vi "test map utils.vi"() -> (2 "pass?":bool)   [LabVIEW 2019, in "LVCOOOP Tests.lvlib"]
uses:
  LVCOOOP Tests.lvlib
  8b7a900f-a1a1-466e-ab71-210356f2434b.vi
  190aee8e-c763-49bc-a4e3-4cdfa35dd57b.vi
  96190adf-c521-424e-a970-e60fe1e5d14e.vi
  571cc04a-834a-4641-954f-49a22e815eb4.vi
  8aebfca1-6881-489a-a878-9dc2cedf487c.vi
  190aee8e-c763-49bc-a4e3-4cdfa35dd57b.vi/c8492b05-ff29-40b2-a5ff-33168be8e6c9.vi
  190aee8e-c763-49bc-a4e3-4cdfa35dd57b.vi/526c77d6-d464-474c-8c7e-61fb6c6ee00b.vi
  96190adf-c521-424e-a970-e60fe1e5d14e.vi/578787be-62c6-45bf-87d1-0e9d7abea452.vi
  571cc04a-834a-4641-954f-49a22e815eb4.vi/4fda8e21-d138-4b78-861a-4ecd3fd1a996.vi
  571cc04a-834a-4641-954f-49a22e815eb4.vi/209a09e3-fb89-4529-ac2e-fb73b7804d0b.vi
  8aebfca1-6881-489a-a878-9dc2cedf487c.vi/3c635ff8-6c59-4014-89be-5488e03f39c6.vi
panel:
  out "string?":bool
  out "dbl_value? 2":bool
  out "boolean value?":bool
  out "dbl_value?":bool
  out "sections match?":bool
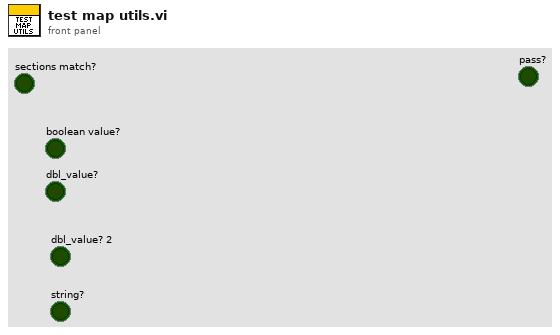
[diagram p1: front panel]
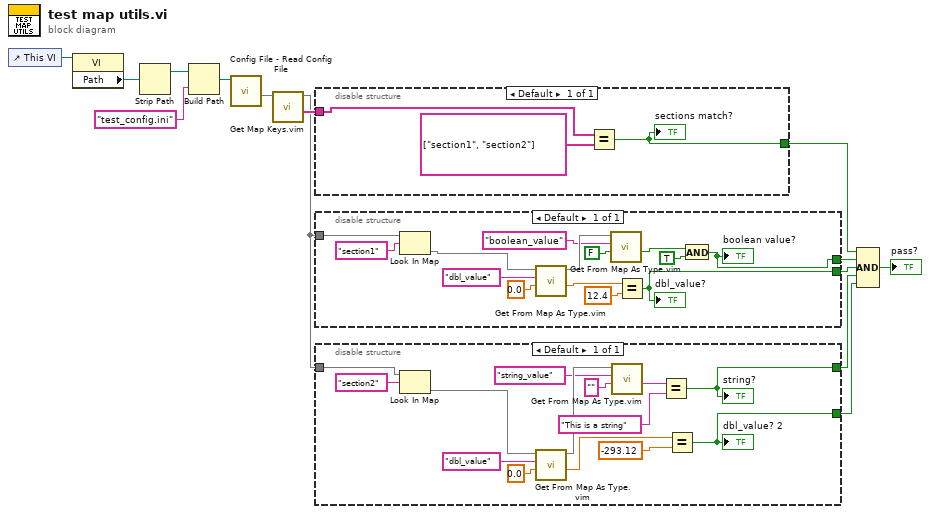
[diagram p0: block diagram]
diagram:
  n1 = control-ref of="This VI"() -> (w14:refnum<vi>)
  n2 = property class="VI"(reference=w14) -> ("Path"=w13:path)  [unwired: 1 in, 2 out]
  n3 = Strip Path(path=w13) -> (stripped path=w12:path)  [unwired: 1 out]
  n4 = Build Path(base path=w12, name or relative path="test_config.ini") -> (appended path=w10:path)
  n5 = call "Config File - Read Config File.vi"("config file path"=w10) -> ("config settings"=w9:map{string, map{string, string}})  [unwired: 9 in, 1 out]
  n6 = call "Get Map Keys.vim"("Map"=w9) -> ("keys"=w8:string[], "Map (dup)"=w7:map{string, map{string, string}})  [unwired: 9 in]
  n7 = disable-structure shown="Default" {
    disable-tunnel: w8 -> [w16]
    disable-tunnel: [w15] -> w6
    frame Enabled {
      n8 = Equal?(x=w16, y=string[] ["section1", "section2"] ("keys")) -> (x = y?=w15:bool)
      "sections match?" <- w15
    }
  }
  n9 = disable-structure shown="Default" {
    disable-tunnel: w7 -> [w20]
    disable-tunnel: [w19] -> w5
    disable-tunnel: [w18] -> w4
    frame Enabled {
      n10 = Look In Map(map=w20, key="section1") -> (value=w30:map{string, string})  [unwired: 1 in, 1 out]
      n11 = call "Get From Map As Type.vim"("default"=0.0, "key"="dbl_value", "map in"=w30) -> ("value"=w27:dbl, "map out (unchanged)"=w25:map{string, string})  [unwired: 5 in, 2 out]
      n12 = call "Get From Map As Type.vim"("default"=FALSE ("dbl_value?"), "key"="boolean_value", "map in"=w25) -> ("value"=w22:bool)  [unwired: 5 in, 3 out]
      n13 = Equal?(x=w27, y=12.4) -> (x = y?=w18:bool)
      "dbl_value?" <- w18
      n14 = And(x=w22, y=TRUE) -> (x .and. y?=w19:bool)
      "boolean value?" <- w19
    }
  }
  n15 = disable-structure shown="Default" {
    disable-tunnel: w7 -> [w44]
    disable-tunnel: [w33] -> w3
    disable-tunnel: [w32] -> w2
    frame Enabled {
      n16 = Look In Map(map=w44, key="section2") -> (value=w43:map{string, string})  [unwired: 1 in, 1 out]
      n17 = call "Get From Map As Type.vim"("default"=0.0, "key"="dbl_value", "map in"=w43) -> ("value"=w39:dbl, "map out (unchanged)"=w42:map{string, string})  [unwired: 5 in, 2 out]
      n18 = call "Get From Map As Type.vim"("default"="" ("key"), "key"="string_value", "map in"=w42) -> ("value"=w35:string)  [unwired: 5 in, 3 out]
      n19 = Equal?(x=w35, y="This is a string" ("key")) -> (x = y?=w33:bool)
      "string?" <- w33
      n20 = Equal?(x=w39, y=-293.12) -> (x = y?=w32:bool)
      "dbl_value? 2" <- w32
    }
  }
  n21 = Compound Arithmetic op=AND(w6, w5, w4, w3, w2) -> (→"pass?":bool)
